vi "Matrix to Raw Data.vi"(11 "Matrix":T1) -> (3 "Raw Data":u8[](array[numeric]))   [LabVIEW 2019, in "LED Matrix Host.lvlib"]
uses:
  LED Matrix Host.lvlib
  Controls/Frame.ctl
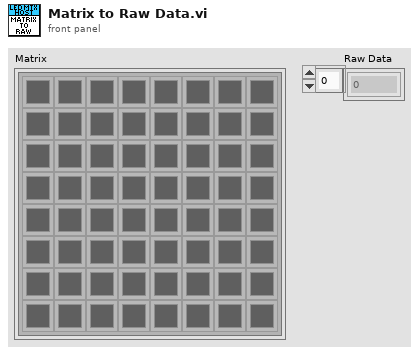
[diagram p1: front panel]
types:
  T1 = typedef "LED Matrix Host.lvlib/Frame.ctl" = cluster{"Matrix":u32[][]}
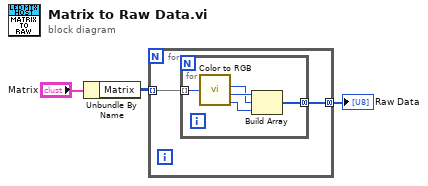
[diagram p0: block diagram]
diagram:
  n1 = Unbundle By Name("Matrix") -> ("Matrix"=w2:u32[][])
  n2 = for {
    tunnel: w2 -> [w5] mode=indexing
    tunnel: [w4] -> w1 mode=concatenating
    n3 = for {
      tunnel: w5 -> [w10] mode=indexing
      tunnel: [w6] -> w4 mode=concatenating
      n4 = call <vilib>:"Color to RGB.vi"("Color"=w10) -> ("R"=w8:u8, "G"=w9:u8, "B"=w7:u8)  [unwired: 1 out]
      n5 = Build Array(w9, w8, w7) -> (w6:u8[])
    }
  }
  "Raw Data" <- w1
